vi "Parsing variable data--With Alias.vi"(8 "error in (no error)":errorcluster, 10 "data":string[][](array[string]), 11 "SQL Server Info":T2) -> (0 "error out":errorcluster, 3 "appended array":string[](array[string]))   [LabVIEW 2020]
doc: "This subvi parse the database variable nformation to controls\nInput\n1. SQL server info\n2. Error in\nOutput\n1. Array (Parsed Data in cluster format)\n2. Error out"
uses:
  Shared/MySQL/typedefs/mysql_authentication.ctl
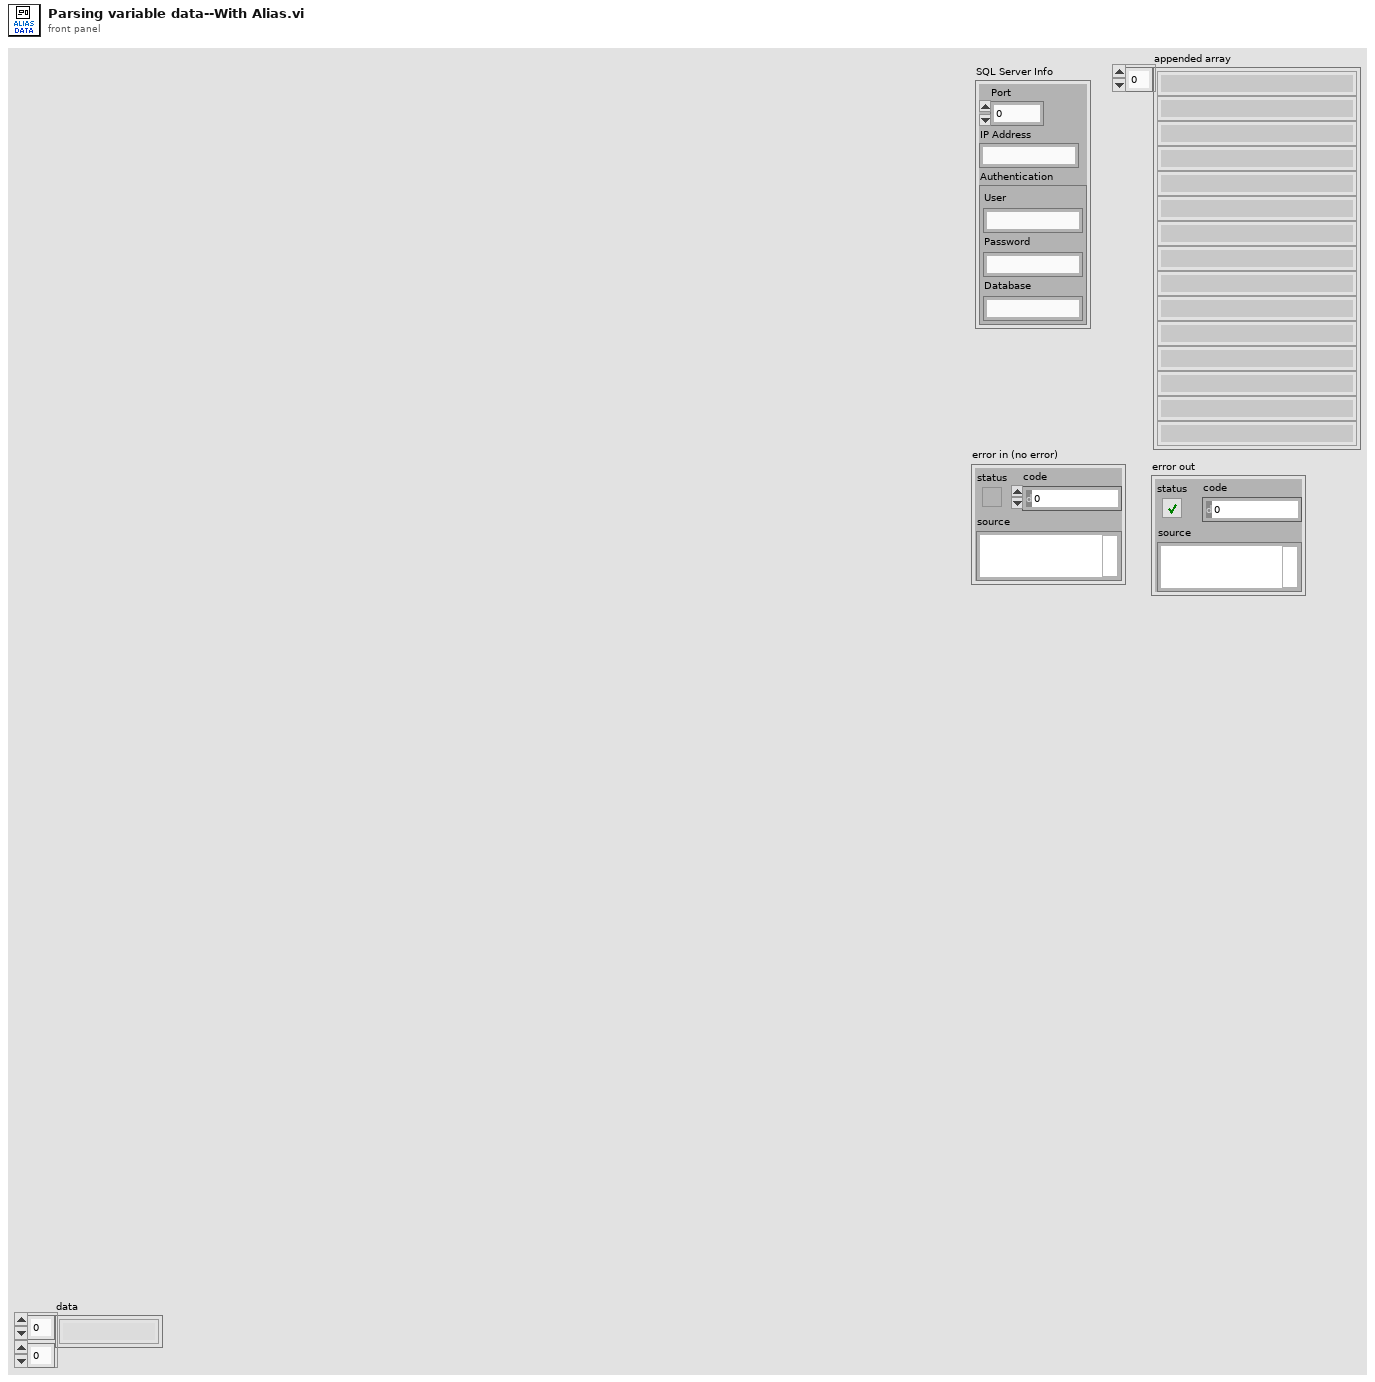
[diagram p1: front panel]
types:
  T1 = typedef "mysql_authentication.ctl" = cluster{"User":string, "Password":string, "Database":string}
  T2 = cluster{"Port":u16, "IP Address":string, "Authentication":T1}
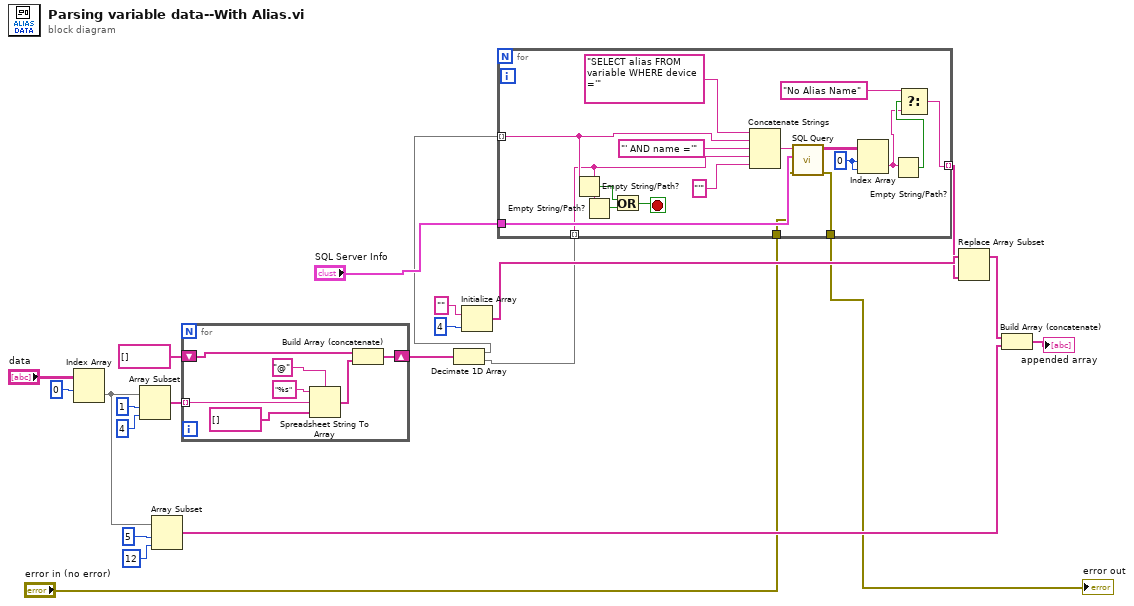
[diagram p0: block diagram]
diagram:
  n1 = Index Array(array="data", index (row)=0) -> (element=w16:string[])  [unwired: 1 in]
  n2 = Array Subset(array=w16, index=1, length=4) -> (w11:string[])
  n3 = Array Subset(array=w16, index=5, length=12) -> (w19:string[])
  n4 = for {
    tunnel: w11 -> [w27] mode=indexing
    shift-right: [w24] -> w13
    shift-left: string[] [] -> [w26]
    n5 = Spreadsheet String To Array(delimiter (Tab)="@", format string="%s", spreadsheet string=w27, array type (2D Dbl)=string[] []) -> (array=w25:string[])
    n6 = Build Array (concatenate)(w26, w25) -> (w24:string[])
  }
  n7 = Decimate 1D Array(w13) -> (w5:string[], w4:string[])
  n8 = Initialize Array("", 4 ("dimension size")) -> (w21:string[])
  n9 = for {
    tunnel: "SQL Server Info" -> [w44]
    tunnel: w5 -> [w38] mode=indexing
    tunnel: w4 -> [w37] mode=indexing
    tunnel: [w30] -> w3 mode=indexing
    tunnel: "error in (no error)" -> [w36]
    tunnel: [w35] -> w1
    stop <- w39 stop-if-true
    w43 = 0 ("disabled index (col)")
    n10 = Empty String/Path?(string/path=w38) -> (empty?=w41:bool)
    n11 = Empty String/Path?(string/path=w37) -> (empty?=w40:bool)
    n12 = Or(x=w41, y=w40) -> (x .or. y?=w39:bool)
    n13 = Concatenate Strings("SELECT alias FROM variable WHERE device ='", w38, "' AND name ='" ("string"), w37, "'" ("string")) -> (w45:string)
    n14 = call "SQL Query.vi"("error in (no error)"=w36, "SQL Server Info"=w44, "Query"=w45) -> ("error out"=w35:errorcluster, "data"=w42:string[][])  [unwired: 7 in]
    n15 = Index Array(array=w42, index (row)=w43, index (col)=w43) -> (element=w31:string)
    n16 = Empty String/Path?(string/path=w31) -> (empty?=w33:bool)
    n17 = Select(t="No Alias Name" ("string"), s=w33, f=w31) -> (s? t:f=w30:string)
  }
  "error out" <- w1
  n18 = Replace Array Subset(array=w21, new element=w3) -> (w22:string[])  [unwired: 1 in]
  n19 = Build Array (concatenate)(w22, w19) -> (→"appended array":string[])
